vi "SetTemp.vi"(9 "Temp C":string="BONTS-82-Temp_C_Input", 10 "Temp B":string="BONTS-82-Temp_B_Input", 11 "Temp A":string="BONTS-82-Temp_A_Input") -> (0 "error out":errorcluster)   [LabVIEW 2021]
uses:
  <vilib>/DAQmx/write.llb/DAQmx Write (Analog DBL 1Chan 1Samp).vi
  <vilib>/DAQmx/miscellaneous.llb/DAQmx Fill In Error Info.vi
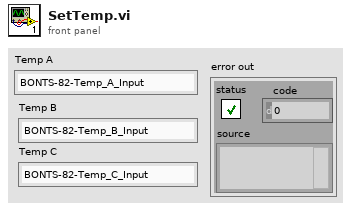
[diagram p1: front panel]
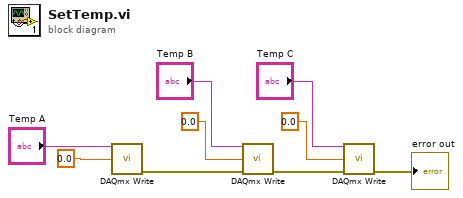
[diagram p0: block diagram]
diagram:
  n1 = call-poly <vilib>:"DAQmx Write.vi"("task/channels in"="Temp A", "data"=0.0) -> ("error out"=w9:errorcluster)  [unwired: 11 in, 2 out]
  n2 = call-poly <vilib>:"DAQmx Write.vi"("task/channels in"="Temp B", "data"=0.0, "error in"=w9) -> ("error out"=w8:errorcluster)  [unwired: 10 in, 2 out]
  n3 = call-poly <vilib>:"DAQmx Write.vi"("task/channels in"="Temp C", "data"=0.0, "error in"=w8) -> ("error out"=→"error out":errorcluster)  [unwired: 10 in, 2 out]
